vi "Equals.vi"(10 "Keyname":refnum<class "Key Name.lvclass">, 11 "Keyname in":refnum<class "Key Name.lvclass">) -> (2 "Equal?":bool, 3 "Keyname out":refnum<class "Key Name.lvclass">)   [LabVIEW 2024, in "Electronic Datasheet.lvlib" / "Key Name.lvclass"]
doc: "checks for equality in the CANopen sense"
uses:
  Key Name.lvclass
  Key Name.lvclass/Key Name.ctl
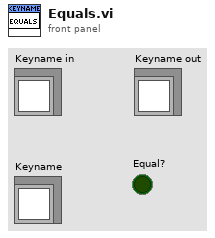
[diagram p1: front panel]
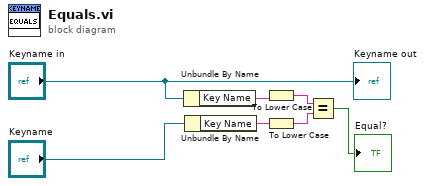
[diagram p0: block diagram]
diagram:
  n1 = Unbundle By Name("Keyname in") -> ("Key Name"=w5:string)
  n2 = Unbundle By Name("Keyname") -> ("Key Name"=w4:string)
  n3 = To Lower Case(string=w5) -> (all lower case string=w2:string)
  n4 = To Lower Case(string=w4) -> (all lower case string=w3:string)
  n5 = Equal?(x=w2, y=w3) -> (x = y?=→"Equal?":bool)
  "Keyname out" <- "Keyname in"
